vi "数据传输.vi"() -> ()   [LabVIEW 2021]
panel:
  in  "布尔":bool
  out "温度曲线":waveform(dbl)[](graph)
  out "数据":waveform(dbl)[](array[waveform])
  out "温度情况":string[][](table)
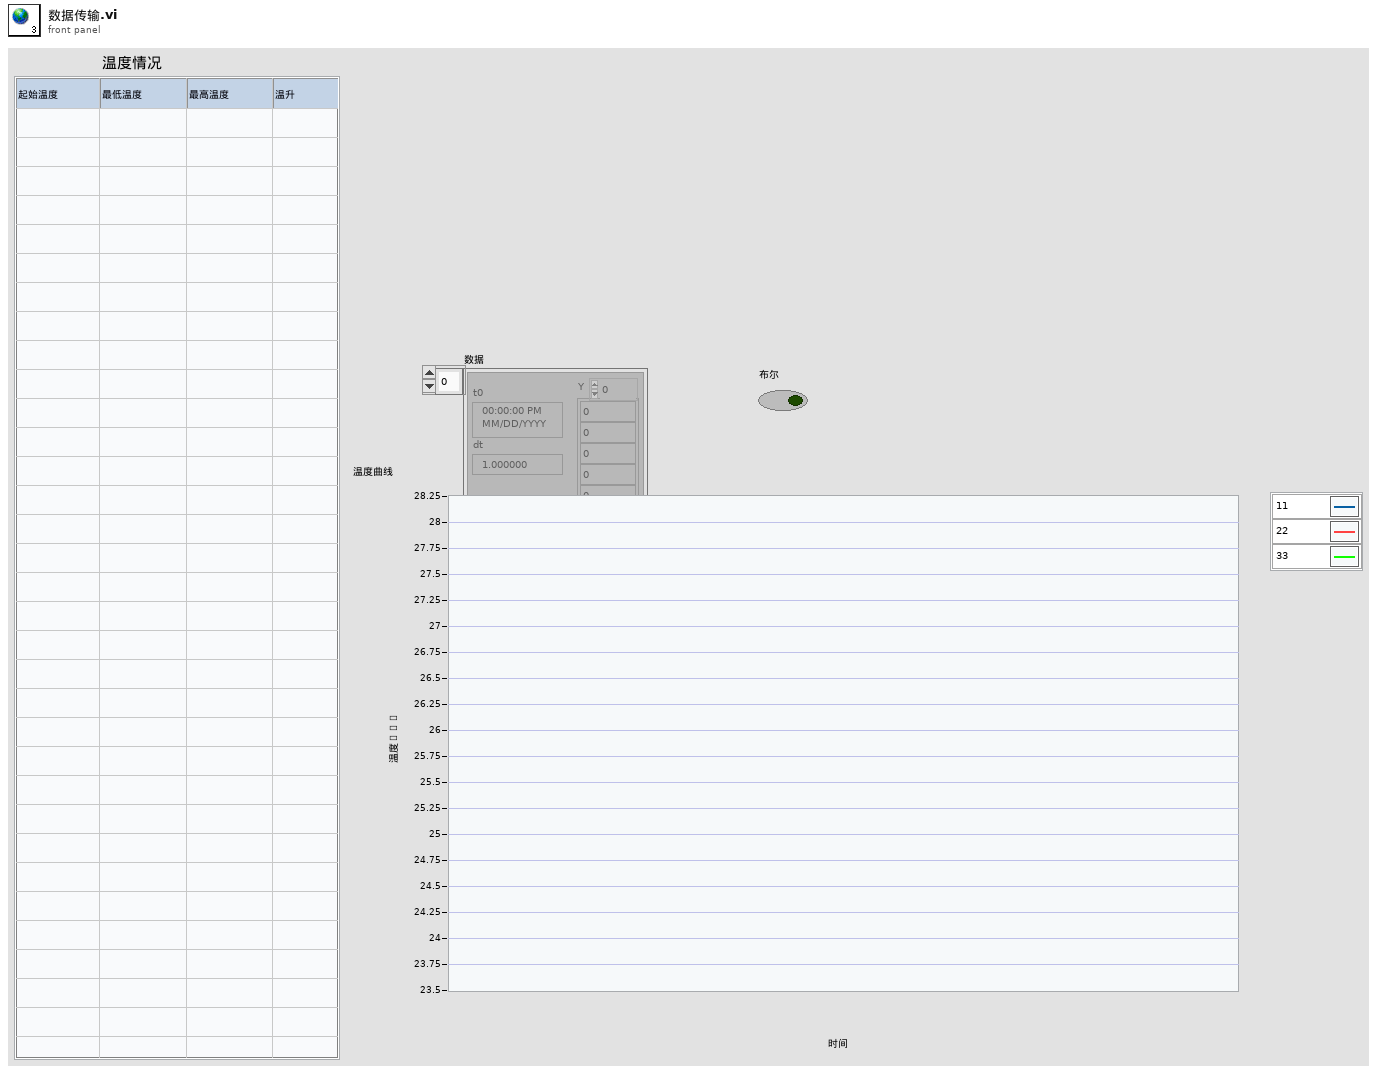
[diagram p1: front panel]
diagram:
